vi "Currents Set.vi"(8 "error in":errorcluster, 10 "Cluster":T1) -> (0 "error out":errorcluster)   [LabVIEW 2020, in "YP PowerControl.lvlib"]
doc: "<b>Note</b>: This VI was renamed by the DQMH Rename Event utility. Make sure the VI Description is updated to reflect the new event name, then delete this comment.\n\n\n_____\nCreated using DQMH Event Scripter 6.0.0.122."
uses:
  YP PowerControl.lvlib
  Currents Set Argument--cluster.ctl
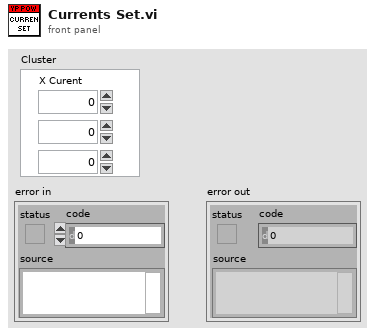
[diagram p1: front panel]
types:
  T1 = cluster{"Z Curent":dbl, "Y Curent":dbl, "X Curent":dbl}
  T2 = typedef "YP PowerControl.lvlib/Currents Set Argument--cluster.ctl" = cluster{"X Curent":dbl, "Y Curent ":dbl, "Z Curent ":dbl}
  T3 = typedef "YP PowerControl.lvlib/Request Events--cluster.ctl" = cluster{"Stop Module":refnum<user-event>, "Show Panel":refnum<user-event>, "Hide Panel":refnum<user-event>, "Get Module Execution Status":refnum<user-event>, "Show Diagram":refnum<user-event>, "Currents Set":refnum<user-event>, "InitializationCommunication":refnum<user-event>}
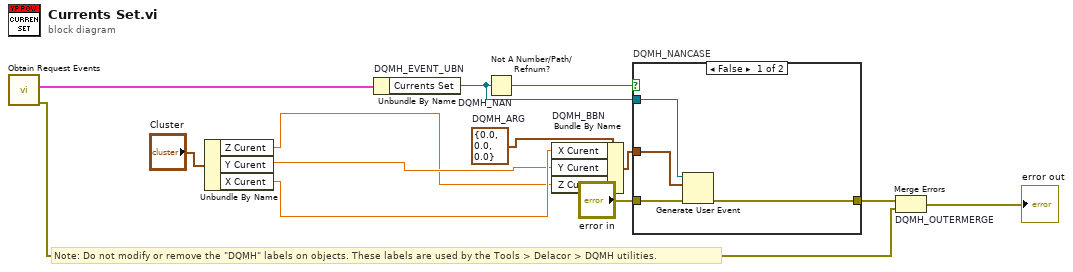
[diagram p0: block diagram]
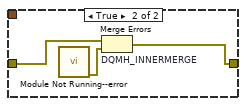
[diagram p2: hidden frame]
diagram:
  w7 = T2 {"X Curent"=0.0, "Y Curent "=0.0, "Z Curent "=0.0}  # DQMH_ARG
  # "Note: Do not modify or remove the \"DQMH\" labels on objects. These labels are used by the Tools > Delacor > DQMH utilities."
  n1 = call "Obtain Request Events.vi"() -> ("error out"=w6:errorcluster, "YP PowerControl Request Events"=w5:T3)  [unwired: 10 in]
  n2 = Unbundle By Name("Cluster") -> ("Z Curent"=w1:dbl, "Y Curent"=w2:dbl, "X Curent"=w3:dbl)
  n3 = Unbundle By Name "DQMH_EVENT_UBN"(w5) -> ("Currents Set"=w9:refnum<user-event>)
  n4 = Not A Number/Path/Refnum? "DQMH_NAN"(number/path/refnum=w9) -> (NaN/Path/Refnum?=w10:bool)
  n5 = Bundle By Name "DQMH_BBN"(cluster=w7, "X Curent"=w3, "Y Curent"=w2, "Z Curent"=w1) -> (w11:T2)
  n6 = case "DQMH_NANCASE" shown="False" w10 {
    tunnel: "error in" -> [w17 w20]
    tunnel: [w16 w19] -> w8
    tunnel: w9 -> [w15 _]
    tunnel: w11 -> [w14 _]
    frame False {
      n7 = Generate User Event(user event=w15, event data cluster=w14, error in=w17) -> (error out=w16:errorcluster)  [unwired: 1 in, 1 out]
    }
    frame True {
      n8 = call "Module Not Running--error.vi"() -> ("error out"=w18:errorcluster)  [unwired: 11 in]
      n9 = Merge Errors "DQMH_INNERMERGE"(w20, w18) -> (w19:errorcluster)
    }
  }
  n10 = Merge Errors "DQMH_OUTERMERGE"(w8, w6) -> (→"error out":errorcluster)
